vi "Append error.vi"(8 "error in (no error)":errorcluster, 9 "error":errorcluster, 10 "code":i32, 11 "Simulated_CCD_Camera in":refnum<class "Simulated_CCD_Camera.lvclass">) -> (0 "error out":errorcluster, 3 "Simulated_CCD_Camera out":refnum<class "Simulated_CCD_Camera.lvclass">)   [LabVIEW 2018, in "Simulated_CCD_Camera.lvclass"]
doc: "Append an error to the array of errors of the class\n\nThis array is verified before the start of an exposure. If an error is found, the exposure will not occur."
uses:
  Simulated_CCD_Camera.lvclass
  Simulated_CCD_Camera.lvclass/Simulated_CCD_Camera.ctl
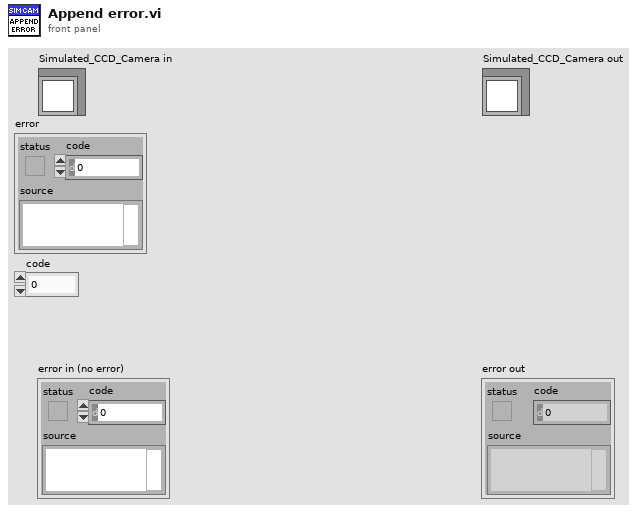
[diagram p1: front panel]
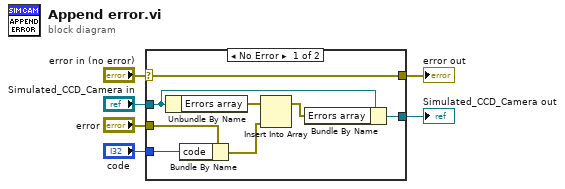
[diagram p0: block diagram]
diagram:
  n1 = case shown="No Error" "error in (no error)" {
    selector: "error in (no error)" -> [w14 w16]
    tunnel: [w14 w16] -> w5
    tunnel: [w11 w15] -> w3
    tunnel: "Simulated_CCD_Camera in" -> [w12 w15]
    tunnel: "error" -> [w8 _]
    tunnel: "code" -> [w7 _]
    frame No Error {
      n2 = Unbundle By Name(w12) -> ("Errors array"=w13:errorcluster[])
      n3 = Bundle By Name(cluster=w8, "code"=w7) -> (w9:errorcluster)
      n4 = Insert Into Array(array=w13, new element=w9) -> (w10:errorcluster[])  [unwired: 1 in]
      n5 = Bundle By Name(cluster=w12, "Errors array"=w10) -> (w11:refnum<class "Simulated_CCD_Camera.lvclass">)
    }
    frame Error {
    }
  }
  "error out" <- w5
  "Simulated_CCD_Camera out" <- w3
